vi "Keithley 2002 Calc3 Config.vi"(0 "GPIB address":string="16", 2 "upper limit 1":dbl=1.0 step=1.0 format="%.6e", 3 "lower limit 1":dbl=-1.0 step=1.0 format="%.6e", 4 "UL1 fail line":dbl min=0.0 max=15.0 step=1.0, 5 "limit 1 test":bool, 6 "LL1 fail line":dbl min=0.0 max=15.0 step=1.0, 7 "limit 2 test":bool, 8 "UL2 fail line":dbl min=0.0 max=15.0 step=1.0, 9 "pass line":dbl min=0.0 max=15.0 step=1.0, 10 "LL2 fail line":dbl min=0.0 max=15.0 step=1.0, 11 "error in":T1, 12 "binning strobe":bool, 13 "upper limit 2":dbl=1.0 step=1.0 format="%.6e", 14 "lower limit 2":dbl=-1.0 step=1.0 format="%.6e") -> (15 "error out":T1)   [LabVIEW 2020]
doc: "This VI is used to configure the settings for math calculation 3. This involves performing limit tests on each measurement.\n\nTo read the results of the calculation, use the Calc Read VI."
panel:
  # "on\noff"
  # "on\noff"
  # "on\noff"
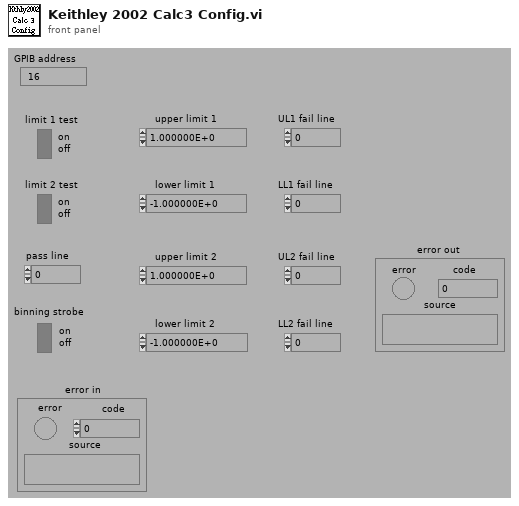
[diagram p1: front panel]
types:
  T1 = cluster{"error":bool, "code":i32, "source":string}
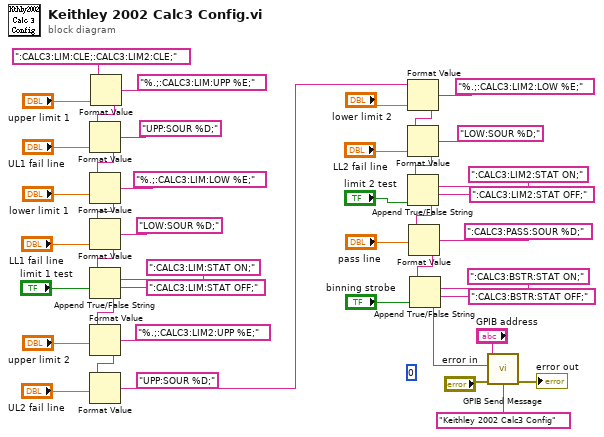
[diagram p0: block diagram]
diagram:
  (unwired) 0
  n1 = Format Value(string ("")=":CALC3:LIM:CLE;:CALC3:LIM2:CLE;", format string="%.;:CALC3:LIM:UPP %E;", value (0)="upper limit 1") -> (output string=w36:string)
  n2 = Format Value(string ("")=w36, format string="UPP:SOUR %D;", value (0)="UL1 fail line") -> (output string=w30:string)
  n3 = Format Value(string ("")=w30, format string="%.;:CALC3:LIM:LOW %E;", value (0)="lower limit 1") -> (output string=w35:string)
  n4 = Format Value(string ("")=w35, format string="LOW:SOUR %D;", value (0)="LL1 fail line") -> (output string=w26:string)
  n5 = Append True/False String(1:"limit 1 test", 2:":CALC3:LIM:STAT OFF;", 3:":CALC3:LIM:STAT ON;", 4:w26) -> (0:w22:string)
  n6 = Format Value(string ("")=w22, format string="%.;:CALC3:LIM2:UPP %E;", value (0)="upper limit 2") -> (output string=w24:string)
  n7 = Format Value(string ("")=w24, format string="UPP:SOUR %D;", value (0)="UL2 fail line") -> (output string=w14:string)
  n8 = Format Value(string ("")=w14, format string="%.;:CALC3:LIM2:LOW %E;", value (0)="lower limit 2") -> (output string=w15:string)
  n9 = Format Value(string ("")=w15, format string="LOW:SOUR %D;", value (0)="LL2 fail line") -> (output string=w10:string)
  n10 = Append True/False String(1:"limit 2 test", 2:":CALC3:LIM2:STAT OFF;", 3:":CALC3:LIM2:STAT ON;", 4:w10) -> (0:w7:string)
  n11 = Format Value(string ("")=w7, format string=":CALC3:PASS:SOUR %D;", value (0)="pass line") -> (output string=w4:string)
  n12 = Append True/False String(1:"binning strobe", 2:":CALC3:BSTR:STAT OFF;", 3:":CALC3:BSTR:STAT ON;", 4:w4) -> (0:w3:string)
  n13 = call "GPIB Send Message.vi"("address string"="GPIB address", "write buffer"=w3, "source"="Keithley 2002 Calc3 Config", "error in"="error in") -> ("error out"=→"error out":T1)  [unwired: 3 in, 2 out]
